vi "Stop Core.vi"(10 "final error code":i32, 11 "Customer in":refnum<class "Customer.lvclass">) -> (3 "Customer out":refnum<class "Customer.lvclass">)   [LabVIEW 2023, in "Customer.lvlib" / "Customer.lvclass"]
doc: "(<B>Filename</B>: Actor Framework.lvlib:Actor.lvclass:Stop Core.vi)\n\nDefines what the actor does before it stops. Use the <B>final error code</B> input to determine whether the actor shut down in response to an error.\n\nBy default, this method does nothing. A descendant class may override it to define behavior, such as shutting down any processes the actor initiated in its override of the Actor Core method."
uses:
  Customer.lvclass
  Customer.lvclass/Customer.ctl
  Person/Person.lvclass
panel:
  out "error out":errorcluster
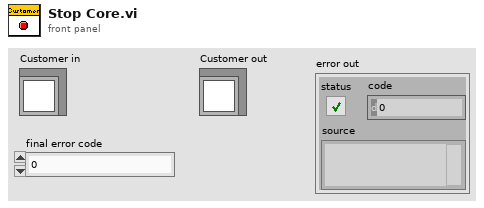
[diagram p1: front panel]
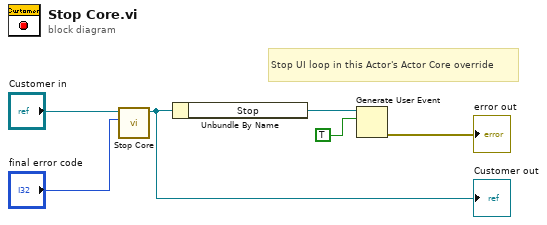
[diagram p0: block diagram]
diagram:
  # "Stop UI loop in this Actor's Actor Core override"
  n1 = call-parent "Stop Core.vi"("final error code"="final error code", "Person in"="Customer in") -> ("Person out"=w2:refnum<class "Customer.lvclass">)  [unwired: 9 in]
  "Customer out" <- w2
  n2 = Unbundle By Name(w2) -> ("Stop"=w4:refnum<user-event>)
  n3 = Generate User Event(user event=w4, event data cluster=TRUE ("event data")) -> (error out=→"error out":errorcluster)  [unwired: 2 in, 1 out]
